vi "Express Harmonic Distortion .vi"(0 "signal in":waveform(dbl)[](array[waveform]), 1 "stop search at Nyquist":bool=TRUE, 5 "export signals":T1(ring)=enum."fundamental signal", 7 "approx. fund. freq. (optional)":dbl=-1.0 format="%0.2p", 9 "highest harmonic":i32=19, 11 "error in (no error)":errorcluster, 12 "search (+/- % of fund.)":dbl=5.0 format="%0.2p") -> (3 "exported spectrum (dB)":waveform(dbl)[](graph), 4 "detected fundamental frequency":waveform(dbl)[](graph), 6 "THD":waveform(dbl)[](graph), 10 "components level":dbl[][](array[numeric]) format="%0.3p", 14 "exported time signal":waveform(dbl)[](graph), 15 "error out":errorcluster)   [LabVIEW 2020]
uses:
  <vilib>/measure/matone.llb/Harmonic Distortion Analyzer 1 Chan.vi
  <vilib>/measure/NI_MAPro.lvlib
panel:
  # "Harmonic Distortion\nAnalyzer"
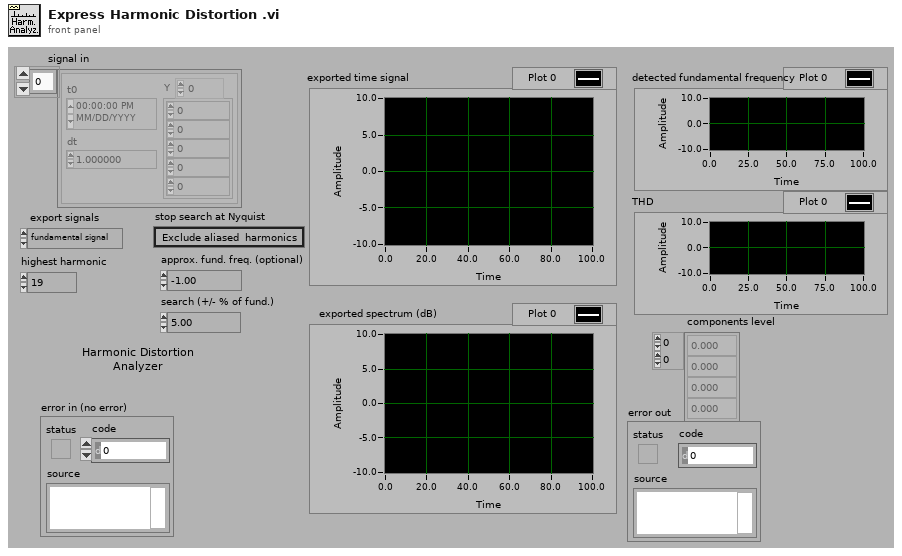
[diagram p1: front panel]
types:
  T1 = enum16{"none", "input signal", "fundamental signal", "residual signal", "harmonics only"}
  T2 = cluster{"approx. fund. freq. (optional)":dbl, dbl}
  T3 = cluster{"exported time signal":waveform(dbl), "exported spectrum (dB)":cluster{"f0":dbl, "df":dbl, "dB Spectrum (Hann)":dbl[]}}
  T4 = cluster{"f0":dbl, "df":dbl, "dB Spectrum (Hann)":dbl[]}
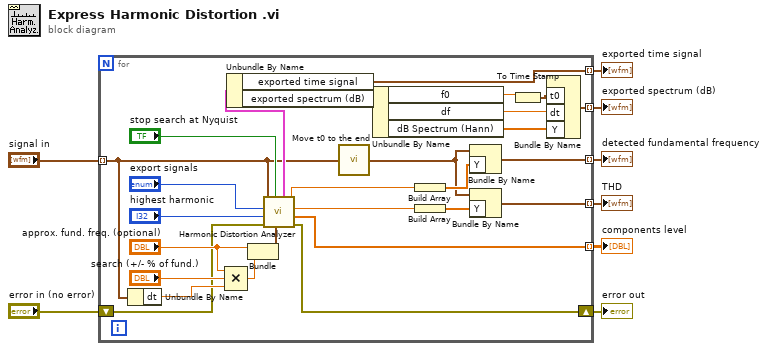
[diagram p0: block diagram]
diagram:
  n1 = for {
    tunnel: "signal in" -> [w14] mode=indexing
    tunnel: [w31] -> w7 mode=indexing
    tunnel: [w30] -> w6 mode=indexing
    tunnel: [w26] -> w5 mode=indexing
    tunnel: [w25] -> w4 mode=indexing
    tunnel: [w22] -> w3 mode=indexing
    shift-right: [w15] -> w2
    shift-left: "error in (no error)" -> [w16]
    n2 = Unbundle By Name(w14) -> ("dt"=w19:dbl)
    n3 = Compound Arithmetic op=MULTIPLY("approx. fund. freq. (optional)", "search (+/- % of fund.)", w19) -> (w18:dbl)
    n4 = Bundle("approx. fund. freq. (optional)"="approx. fund. freq. (optional)", w18) -> (w29:T2)  [unwired: 1 in]
    n5 = call-poly <vilib>:"Harmonic Distortion Analyzer.vi"("advanced search"=w29, "stop search at Nyquist"="stop search at Nyquist", "error in (no error)"=w16, "highest harmonic"="highest harmonic", "export mode"="export signals", "signal in"=w14) -> ("error out"=w15:errorcluster, "components level"=w22:dbl[], "THD"=w23:dbl, "detected fundamental frequency"=w24:dbl, "exported signals"=w32:T3)  [unwired: 1 out]
    n6 = Unbundle By Name(w32) -> ("exported time signal"=w31:waveform(dbl), "exported spectrum (dB)"=w12:T4)
    n7 = call <vilib>:"Move t0 to the end.vi"("waveform in"=w14) -> ("waveform out"=w13:waveform(dbl))
    n8 = Unbundle By Name(w12) -> ("f0"=w11:dbl, "df"=w10:dbl, "dB Spectrum (Hann)"=w9:dbl[])
    n9 = Build Array(w24) -> (w28:dbl[])
    n10 = Build Array(w23) -> (w27:dbl[])
    n11 = Bundle By Name(cluster=w13, "Y"=w28) -> (w26:waveform(dbl))
    n12 = Bundle By Name(cluster=w13, "Y"=w27) -> (w25:waveform(dbl))
    n13 = To Time Stamp(1:w11) -> (0:w17:timestamp)
    n14 = Bundle By Name("t0"=w17, "dt"=w10, "Y"=w9) -> (w30:waveform(dbl))  [unwired: 1 in]
  }
  "exported time signal" <- w7
  "exported spectrum (dB)" <- w6
  "detected fundamental frequency" <- w5
  "THD" <- w4
  "components level" <- w3
  "error out" <- w2
